vi "createSavingPath.vi"(1 "pathIn":path=path "C:/temp/test.txt") -> (0 "pathOut":path)   [LabVIEW 2021]
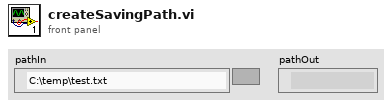
[diagram p1: front panel]
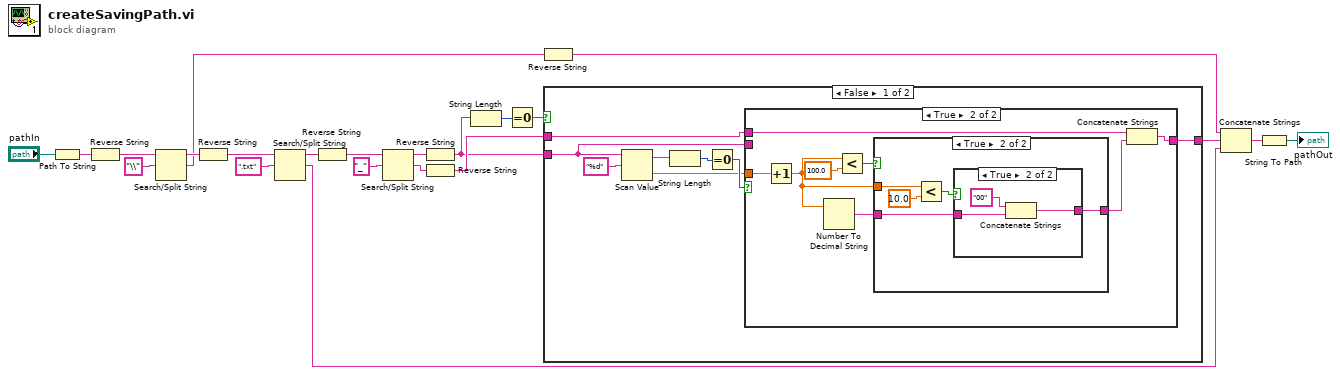
[diagram p0: block diagram]
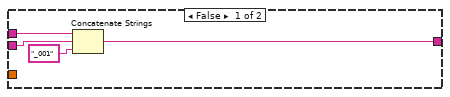
[diagram p2: hidden frame]
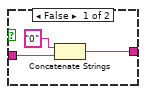
[diagram p4: hidden frame]
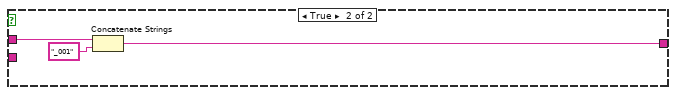
[diagram p5: hidden frame]
diagram:
  n1 = Path To String(path="pathIn") -> (string=w20:string)
  n2 = Reverse String(1:w20) -> (0:w19:string)
  n3 = Search/Split String(string=w19, search string/char (-)="\\") -> (substring before match=w18:string, match + rest of string=w17:string)  [unwired: 1 in, 1 out]
  n4 = Reverse String(1:w18) -> (0:w15:string)
  n5 = Search/Split String(string=w15, search string/char (-)=".txt") -> (substring before match=w8:string, match + rest of string=w13:string)  [unwired: 1 in, 1 out]
  n6 = Reverse String(1:w8) -> (0:w7:string)
  n7 = Search/Split String(string=w7, search string/char (-)="_") -> (substring before match=w4:string, match + rest of string=w6:string)  [unwired: 1 in, 1 out]
  n8 = Reverse String(1:w4) -> (0:w3:string)
  n9 = Reverse String(1:w6) -> (0:w5:string)
  n10 = String Length(string=w3) -> (length=w11:i32)
  n11 = Equal To 0?(x=w11) -> (x = 0?=w10:bool)
  n12 = Reverse String(1:w17) -> (0:w14:string)
  n13 = case shown="False" w10 {
    tunnel: w5 -> [w25 w57]
    tunnel: [w24 w55] -> w9
    tunnel: w3 -> [w23 _]
    frame False {
      n14 = Scan Value(string=w23, format string="%d") -> (output string=w29:string, value=w26:dbl)  [unwired: 1 in]
      n15 = String Length(string=w29) -> (length=w28:i32)
      n16 = Equal To 0?(x=w28) -> (x = 0?=w27:bool)
      n17 = case shown="True" w27 {
        tunnel: w26 -> [_ w42]
        tunnel: w25 -> [w32 w37]
        tunnel: [w33 w35] -> w24
        tunnel: w23 -> [w31 _]
        frame False {
          n18 = Concatenate Strings(w32, w31, "_001" ("string")) -> (w33:string)
        }
        frame True {
          n19 = Increment(x=w42) -> (x+1=w38:dbl)
          n20 = Number To Decimal String(number=w38) -> (decimal integer string=w39:string)  [unwired: 1 in]
          n21 = Less?(x=w38, y=100.0) -> (x < y?=w40:bool)
          n22 = case shown="True" w40 {
            tunnel: w39 -> [w43 w47]
            tunnel: [w43 w48] -> w36
            tunnel: w38 -> [_ w46]
            frame False {
            }
            frame True {
              n23 = Less?(x=w46, y=10.0) -> (x < y?=w44:bool)
              n24 = case shown="True" w44 {
                tunnel: [w51 w52] -> w48
                tunnel: w47 -> [w50 w53]
                frame False {
                  n25 = Concatenate Strings("0" ("string"), w50) -> (w51:string)
                }
                frame True {
                  n26 = Concatenate Strings("00" ("string"), w53) -> (w52:string)
                }
              }
            }
          }
          n27 = Concatenate Strings(w37, w36) -> (w35:string)
        }
      }
    }
    frame True {
      n28 = Concatenate Strings(w57, "_001" ("string")) -> (w55:string)
    }
  }
  n29 = Concatenate Strings(w14, w9, w13) -> (w2:string)
  n30 = String To Path(string=w2) -> (path=→"pathOut":path)
